vi "CLD 6 CSV file utility.vi"(8 "Error In":errorcluster, 9 "name or relative path":string, 10 "[Data In]":T2[](array[typedef])=[{"Step Time Target"=3, "Step 1"=TRUE, "Step 2"=FALSE, "Step 3"=FALSE}, {"Step Time Target"=4, "Step 1"=FALSE, "Step 2"=TRUE, "Step 3"=FALSE}, {"Step Time Target"=5, "Step 1"=FALSE, "Step 2"=FALSE, "Step 3"=TRUE}], 11 "CSV File Enum":T1) -> (0 "Error Out":errorcluster, 3 "[Data Out]":T2[](array[typedef]))   [LabVIEW 2018]
doc: "CLD 6 exercise"
uses:
  CLD 10 CSV file data structure.ctl
  CLD 10 CSV file enum.ctl
  <vilib>/Utility/file.llb/Read Delimited Spreadsheet (string).vi
  <vilib>/Utility/file.llb/Write Delimited Spreadsheet (string).vi
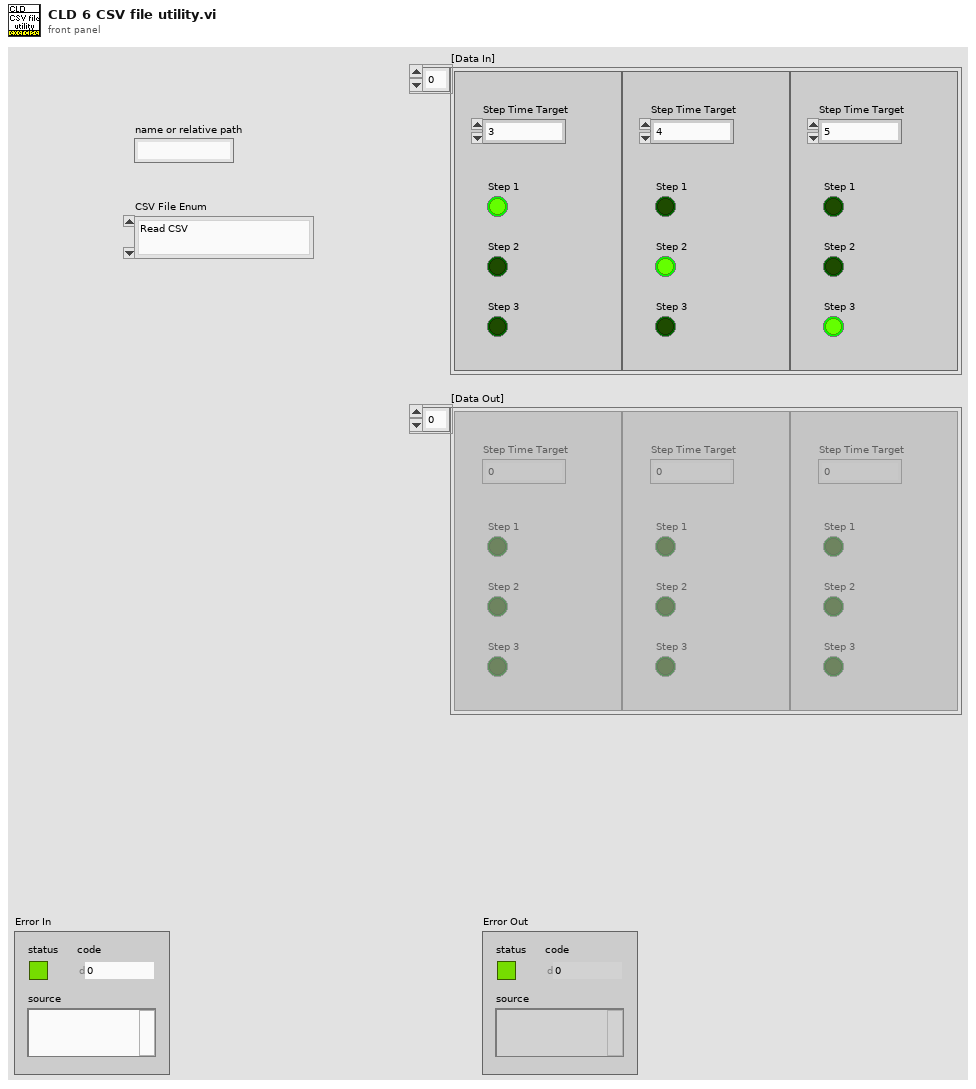
[diagram p1: front panel]
types:
  T1 = typedef "CLD 10 CSV file enum.ctl" = enum16{"Read CSV", "Write CSV"}
  T2 = typedef "CLD 10 CSV file data structure.ctl" = cluster{"Step Time Target":i32, "Step 1":bool, "Step 2":bool, "Step 3":bool}
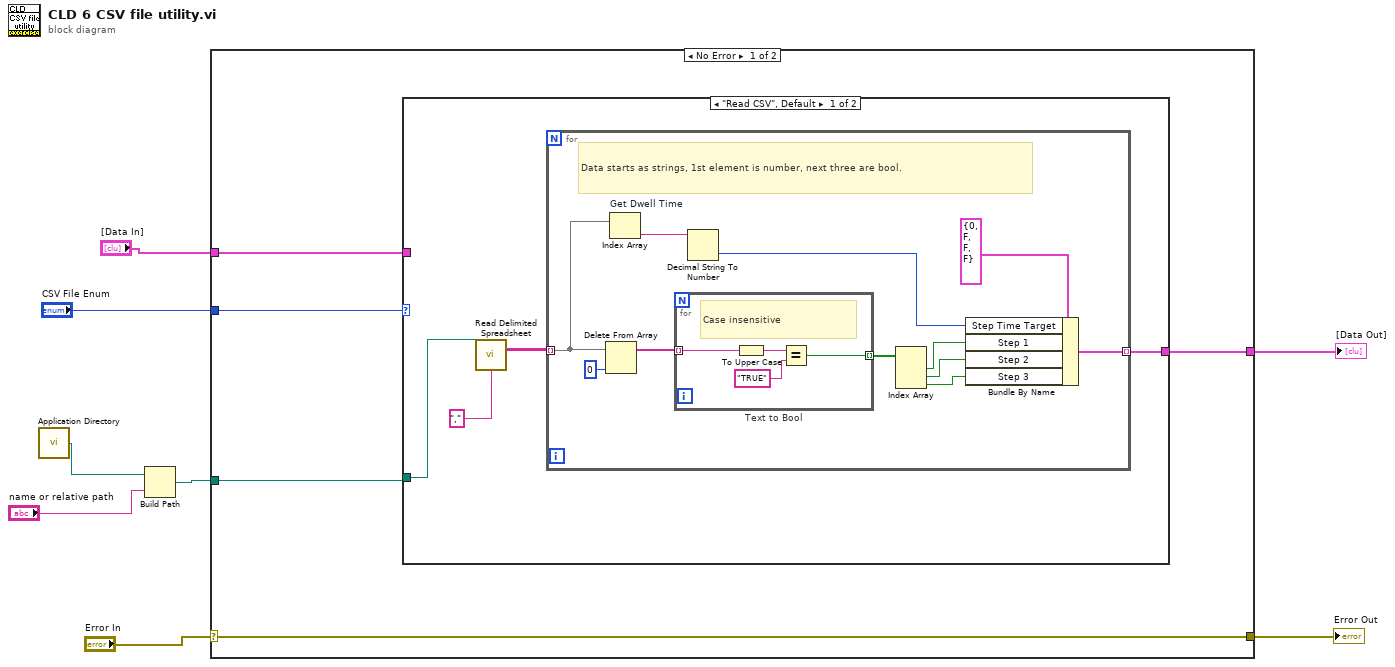
[diagram p0: block diagram]
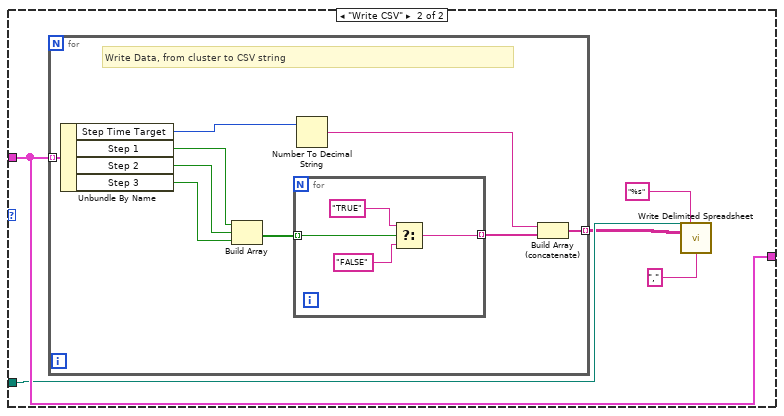
[diagram p2: hidden frame]
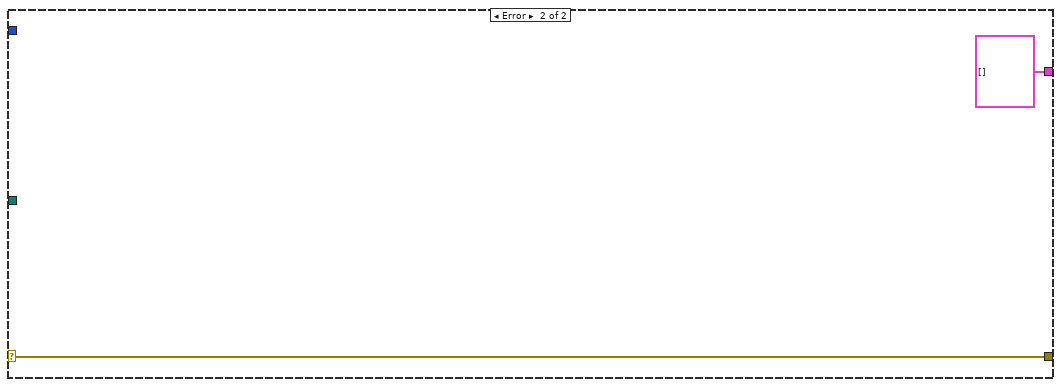
[diagram p3: hidden frame]
diagram:
  n1 = call <vilib>:"Application Directory.vi"() -> ("Application Directory"=w2:path)
  n2 = Build Path(base path=w2, name or relative path="name or relative path") -> (appended path=w3:path)
  n3 = case shown="No Error" "Error In" {
    selector: "Error In" -> [w10 w52]
    tunnel: [w13 T2[] [] ("[Data In]")] -> w7
    tunnel: "CSV File Enum" -> [w12 _]
    tunnel: "[Data In]" -> [w11 _]
    tunnel: [w10 w52] -> w5
    tunnel: w3 -> [w9 _]
    frame No Error {
      n4 = case shown="\"Read CSV\", Default" w12 {
        tunnel: w9 -> [w15 w35]
        tunnel: [w17 w37] -> w13
        tunnel: w11 -> [_ w37]
        frame "Read CSV", Default {
          n5 = call-poly <vilib>:"Read Delimited Spreadsheet.vi"("file path (dialog if empty)"=w15, "delimiter (\\t)"="," ("delimiter (\\t)")) -> ("all rows"=w16:string[][])  [unwired: 8 in, 5 out]
          n6 = for {
            tunnel: w16 -> [w21] mode=indexing
            tunnel: [w28] -> w17 mode=indexing
            # "Data starts as strings, 1st element is number, next three are bool."
            n7 = Delete From Array(array=w21, index=0) -> (array with subset deleted=w19:string[])  [unwired: 1 in, 1 out]
            n8 = Index Array "Get Dwell Time"(array=w21) -> (element=w27:string)  [unwired: 1 in]
            n9 = for "Text to Bool" {
              tunnel: w19 -> [w32] mode=indexing
              tunnel: [w29] -> w25 mode=indexing
              # "Case insensitive"
              n10 = To Upper Case(1:w32) -> (0:w31:string)
              n11 = Equal?(x=w31, y="TRUE") -> (x = y?=w29:bool)
            }
            n12 = Decimal String To Number(string=w27) -> (number=w26:i32)  [unwired: 2 in, 1 out]
            n13 = Index Array(array=w25) -> (element #1=w24:bool, element #2=w23:bool, element #3=w18:bool)  [unwired: 3 in]
            n14 = Bundle By Name(cluster=T2 {"Step Time Target"=0, "Step 1"=FALSE, "Step 2"=FALSE, "Step 3"=FALSE} ("CSV File Data Structure"), "Step Time Target"=w26, "Step 1"=w24, "Step 2"=w23, "Step 3"=w18) -> (w28:T2)
          }
        }
        frame "Write CSV" {
          n15 = for {
            tunnel: w37 -> [w46] mode=indexing
            tunnel: [w38] -> w34 mode=indexing
            # "Write Data, from cluster to CSV string"
            n16 = Unbundle By Name(w46) -> ("Step Time Target"=w45:i32, "Step 1"=w44:bool, "Step 2"=w43:bool, "Step 3"=w42:bool)
            n17 = Build Array(w44, w43, w42) -> (w41:bool[])
            n18 = for {
              tunnel: w41 -> [w50] mode=indexing
              tunnel: [w47] -> w39 mode=indexing
              n19 = Select(t="TRUE", s=w50, f="FALSE") -> (s? t:f=w47:string)
            }
            n20 = Number To Decimal String(number=w45) -> (decimal integer string=w40:string)  [unwired: 1 in]
            n21 = Build Array (concatenate)(w40, w39) -> (w38:string[])
          }
          n22 = call-poly <vilib>:"Write Delimited Spreadsheet.vi"("file path (dialog if empty)"=w35, "format (%s)"="%s", "2D data"=w34, "delimiter (\\t)"="," ("delimiter (\\t)")) -> ()  [unwired: 10 in, 2 out]
        }
      }
    }
    frame Error {
    }
  }
  "[Data Out]" <- w7
  "Error Out" <- w5
